vi "test_get_target_from_id.vi"() -> ()   [LabVIEW 2019]
uses:
  <vilib>/Rock Robotics/WPI/ThirdParty/PhotonVisionLib/TypeDef/PhotonTrackedTargetType.ctl
  <vilib>/Rock Robotics/WPI/ThirdParty/PhotonVisionLib/TypeDef/TargetCornerType.ctl
  <vilib>/Rock Robotics/WPI/ThirdParty/JAS_Junk/TrajLib/TypeDef/TRANSFORM3D.ctl
  <vilib>/Rock Robotics/WPI/ThirdParty/JAS_Junk/TrajLib/TypeDef/TRANSLATION3D.ctl
  <vilib>/Rock Robotics/WPI/ThirdParty/JAS_Junk/TrajLib/TypeDef/ROTATION3D.ctl
  <vilib>/Rock Robotics/WPI/ThirdParty/JAS_Junk/TrajLib/TypeDef/QUATERNION.ctl
  <vilib>/Rock Robotics/WPI/ThirdParty/PhotonVisionLib/SubVI/PhotonPipelineResult_GetLatency_Millis.vi
  <vilib>/Rock Robotics/WPI/ThirdParty/PhotonVisionLib/SubVI/Packet_encode_FLT64.vi
  <vilib>/Rock Robotics/WPI/ThirdParty/PhotonVisionLib/SubVI/Packet_encode_ByteI8.vi
  <vilib>/Rock Robotics/WPI/ThirdParty/PhotonVisionLib/SubVI/PhotonTrackedTarget_Pack.vi
  <vilib>/Rock Robotics/WPI/ThirdParty/PhotonVisionLib/SubVI/PhotonMultiTargetPNPResult_pack.vi
  <vilib>/Rock Robotics/WPI/ThirdParty/PhotonVisionLib/SubVI/Packet_decode_Flt64.vi
  <vilib>/Rock Robotics/WPI/ThirdParty/PhotonVisionLib/SubVI/Packet_decode_ByteI8.vi
  <vilib>/Rock Robotics/WPI/ThirdParty/PhotonVisionLib/SubVI/PhotonTrackedTarget_Unpack.vi
  <vilib>/Rock Robotics/WPI/ThirdParty/PhotonVisionLib/SubVI/PhotonMultiTargetPNPResult_unpack.vi
  <vilib>/Rock Robotics/WPI/ThirdParty/PhotonVisionLib/SubVI/PhotonTrackedTarget_GetArea.vi
  <vilib>/Rock Robotics/WPI/ThirdParty/PhotonVisionLib/SubVI/PhotonTrackedTarget_GetBestCameraToTarget.vi
  <vilib>/Rock Robotics/WPI/ThirdParty/PhotonVisionLib/SubVI/PhotonTrackedTarget_GetMinAreaRectCorners.vi
  <vilib>/Rock Robotics/WPI/ThirdParty/PhotonVisionLib/SubVI/PhotonTrackedTarget_GetPitch.vi
  <vilib>/Rock Robotics/WPI/ThirdParty/PhotonVisionLib/SubVI/PhotonTrackedTarget_GetSkew.vi
  <vilib>/Rock Robotics/WPI/ThirdParty/PhotonVisionLib/SubVI/PhotonTrackedTarget_GetYaw.vi
  <vilib>/Rock Robotics/WPI/ThirdParty/PhotonVisionLib/SubVI/PhotonTrackedTarget_GetAltCameraToTarget.vi
  <vilib>/Rock Robotics/WPI/ThirdParty/PhotonVisionLib/SubVI/Packet_encode_Transform3d.vi
  <vilib>/Rock Robotics/WPI/ThirdParty/PhotonVisionLib/SubVI/PhotonTrackedTarget_GetFiducialId.vi
  <vilib>/Rock Robotics/WPI/ThirdParty/PhotonVisionLib/SubVI/Packet_encode_Int32.vi
  <vilib>/Rock Robotics/WPI/ThirdParty/PhotonVisionLib/SubVI/PhotonTrackedTarget_GetPoseAmbiguity.vi
  <vilib>/Rock Robotics/WPI/ThirdParty/PhotonVisionLib/SubVI/PhotonTrackedTarget_GetDetectedCorners.vi
  <vilib>/Rock Robotics/WPI/ThirdParty/PhotonVisionLib/SubVI/PhotonPNPResult_pack.vi
  <vilib>/Rock Robotics/WPI/ThirdParty/PhotonVisionLib/SubVI/Packet_encode_Int16.vi
  <vilib>/Rock Robotics/WPI/ThirdParty/PhotonVisionLib/SubVI/PhotonMultiTargetPNPResult_MAX_IDS.vi
  <vilib>/Rock Robotics/WPI/ThirdParty/PhotonVisionLib/SubVI/TargetCorner_New.vi
  <vilib>/Rock Robotics/WPI/ThirdParty/PhotonVisionLib/SubVI/Packet_decode_Int32.vi
  <vilib>/Rock Robotics/WPI/ThirdParty/PhotonVisionLib/SubVI/Packet_decode_Transform3d.vi
  <vilib>/Rock Robotics/WPI/ThirdParty/PhotonVisionLib/SubVI/PhotonPNPResult_unpackt.vi
  <vilib>/Rock Robotics/WPI/ThirdParty/PhotonVisionLib/SubVI/PhotonMultiTargetPNPResult_New.vi
  <vilib>/Rock Robotics/WPI/ThirdParty/PhotonVisionLib/SubVI/Packet_decode_Int16.vi
  <vilib>/Rock Robotics/WPI/ThirdParty/JAS_Junk/TrajLib/VI/Transform3d_GetRotation3d.vi
  <vilib>/Rock Robotics/WPI/ThirdParty/JAS_Junk/TrajLib/VI/Transform3d_GetTranslation3d.vi
  <vilib>/Rock Robotics/WPI/ThirdParty/JAS_Junk/TrajLib/VI/Translation3d_ToTranslation2d.vi
  <vilib>/Rock Robotics/WPI/ThirdParty/JAS_Junk/TrajLib/VI/Rotation3d_ToRotation2d.vi
  <vilib>/Rock Robotics/WPI/ThirdParty/JAS_Junk/TrajLib/Transform2d_Create_TransRot.vi
  <vilib>/Rock Robotics/WPI/ThirdParty/JAS_Junk/TrajLib/VI/Transform3d_GetXYZ.vi
  <vilib>/Rock Robotics/WPI/ThirdParty/JAS_Junk/TrajLib/VI/Rotation3d_GetQuaterion.vi
  <vilib>/Rock Robotics/WPI/ThirdParty/JAS_Junk/TrajLib/VI/Quaternion_Get_All.vi
  <vilib>/Rock Robotics/WPI/ThirdParty/PhotonVisionLib/SubVI/Packet_encode_Boolean.vi
  <vilib>/Rock Robotics/WPI/ThirdParty/JAS_Junk/TrajLib/VI/Transform3d_Create_Trans3dRot3d.vi
  <vilib>/Rock Robotics/WPI/ThirdParty/JAS_Junk/TrajLib/VI/Translation3d_Create.vi
  <vilib>/Rock Robotics/WPI/ThirdParty/JAS_Junk/TrajLib/VI/Rotation3d_Create_Quaternion.vi
  <vilib>/Rock Robotics/WPI/ThirdParty/JAS_Junk/TrajLib/VI/Quaternion_New.vi
  <vilib>/Rock Robotics/WPI/ThirdParty/PhotonVisionLib/SubVI/Packet_decode_Boolean.vi
  <vilib>/Rock Robotics/WPI/ThirdParty/PhotonVisionLib/SubVI/PhotonPNPResult_New_Empty.vi
  <vilib>/Rock Robotics/WPI/ThirdParty/PhotonVisionLib/SubVI/PhotonPNPResult_New.vi
  <vilib>/Rock Robotics/WPI/ThirdParty/JAS_Junk/TrajLib/Translation2d_Create.vi
  <vilib>/Rock Robotics/WPI/ThirdParty/JAS_Junk/TrajLib/Rotation2d_CreateAngle.vi
  <vilib>/Rock Robotics/WPI/ThirdParty/JAS_Junk/TrajLib/VI/Rotation3d_GetXYZ.vi
  <vilib>/Rock Robotics/WPI/ThirdParty/JAS_Junk/TrajLib/VI/Translation3d_GetXYZ.vi
  <vilib>/Rock Robotics/WPI/ThirdParty/JAS_Junk/TrajLib/VI/Quaternion_Normalize.vi
  <vilib>/Rock Robotics/WPI/ThirdParty/JAS_Junk/TrajLib/VI/Quaternion_New_Default.vi
  <vilib>/Rock Robotics/WPI/ThirdParty/PhotonVisionLib/PhotonVisionLib.lvlib
  <vilib>/Rock Robotics/WPI/ThirdParty/JAS_Junk/TrajLib/Trajectory_Library.lvlib
panel:
  out "Target Index":i32
  out "Found Target?":bool
  out "PhotonTrackedTarget":T1={"Yaw"=0.0, "Pitch"=0.0, "Area"=0.0, "Skew"=0.0, "MinAreaRectCorners"=[], "BestCameraToTarget"={"TRANSLATION3D"={"X"=0.0, "Y"=0.0, "Z"=0.0}, "ROTATION3D"={"Q_quaternion"={"R"=1.0, "V"=[0.0, 0.0, 0.0]}}, "XF"=FALSE}, "FiiducialId"=0, "AltCameraToTarget"={"TRANSLATION3D"={"X"=0.0, "Y"=0.0, "Z"=0.0}, "ROTATION3D"={"Q_quaternion"={"R"=0.0, "V"=[0.0, 0.0, 0.0]}}, "XF"=FALSE}, "PoseAmbiguity"=0.0, "DetectedCorners"=[]} {"AltCameraToTarget"."TRANSLATION3D"."Z" format="%14.3f"; "AltCameraToTarget"."TRANSLATION3D"."Y" format="%14.3f"; "AltCameraToTarget"."TRANSLATION3D"."X" format="%14.3f"; "BestCameraToTarget"."TRANSLATION3D"."Z" format="%14.3f"; "BestCameraToTarget"."TRANSLATION3D"."Y" format="%14.3f"; "BestCameraToTarget"."TRANSLATION3D"."X" format="%14.3f"}
  in  "ID":i32
  in  "TrackedTargets":T1[](array[typedef]) {"AltCameraToTarget"."TRANSLATION3D"."Z" format="%14.3f"; "AltCameraToTarget"."TRANSLATION3D"."Y" format="%14.3f"; "AltCameraToTarget"."TRANSLATION3D"."X" format="%14.3f"; "BestCameraToTarget"."TRANSLATION3D"."Z" format="%14.3f"; "BestCameraToTarget"."TRANSLATION3D"."Y" format="%14.3f"; "BestCameraToTarget"."TRANSLATION3D"."X" format="%14.3f"}
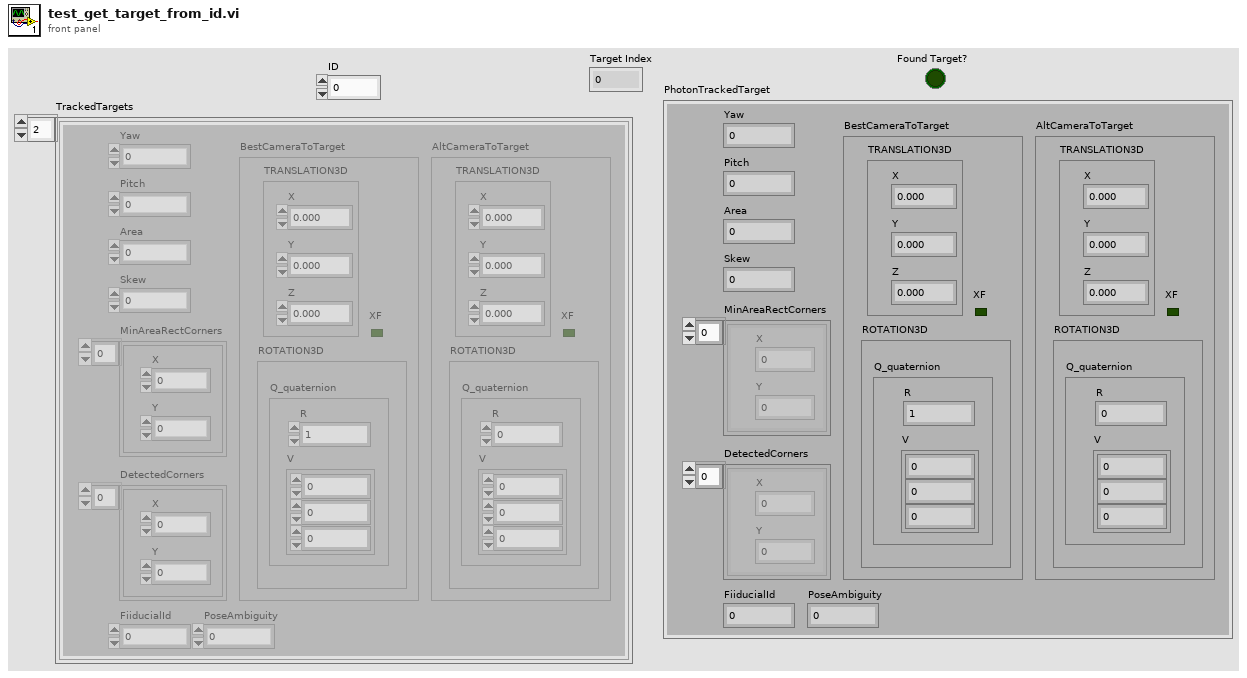
[diagram p1: front panel]
types:
  T1 = typedef "PhotonVisionLib.lvlib/PhotonTrackedTargetType.ctl" = cluster{"Yaw":dbl, "Pitch":dbl, "Area":dbl, "Skew":dbl, "MinAreaRectCorners":T2[], "BestCameraToTarget":T3, "FiiducialId":i32, "AltCameraToTarget":T3, "PoseAmbiguity":dbl, "DetectedCorners":T2[]}
  T2 = typedef "PhotonVisionLib.lvlib/TargetCornerType.ctl" = cluster{"X":dbl, "Y":dbl}
  T3 = typedef "Trajectory_Library.lvlib/TRANSFORM3D.ctl" = cluster{"TRANSLATION3D":T4, "ROTATION3D":T5, "XF":bool}
  T4 = typedef "Trajectory_Library.lvlib/TRANSLATION3D.ctl" = cluster{"X":dbl, "Y":dbl, "Z":dbl}
  T5 = typedef "Trajectory_Library.lvlib/ROTATION3D.ctl" = cluster{"Q_quaternion":T6}
  T6 = typedef "Trajectory_Library.lvlib/QUATERNION.ctl" = cluster{"R":dbl, "V":dbl[]}
  T7 = typedef "PhotonVisionLib.lvlib/PhotonPipelineResultType.ctl" = cluster{"TargetCount":i32, "Latency_MilliSec":dbl, "Targets":T1[], "TimeStampSec":dbl, "PhotonMultiTargetPNPResult":T8}
  T8 = typedef "PhotonVisionLib.lvlib/PhotonMultiTargetPNPResultType.ctl" = cluster{"PhotonPNPResult":T9, "FiducialIDsUsed":i16[]}
  T9 = typedef "PhotonVisionLib.lvlib/PhotonPNPResultType.ctl" = cluster{"IsPresent":bool, "bestReprojErr":dbl, "altReprojErr":dbl, "ambiguity":dbl, "Best":T3, "Alt":T3}
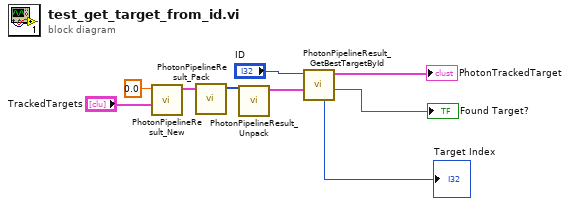
[diagram p0: block diagram]
diagram:
  n1 = call <vilib>:"PhotonPipelineResult_New.vi"("TrackedTargets"="TrackedTargets", "Latency_Millis"=0.0) -> ("PhotonPipelineResult"=w7:T7)  [unwired: 9 in]
  n2 = call <vilib>:"PhotonPipelineResult_Pack.vi"("PhotonPipelineResult"=w7) -> ("Packet_RawData"=w6:u8[])  [unwired: 10 in]
  n3 = call <vilib>:"PhotonPipelineResult_Unpack.vi"("RawData"=w6) -> ("PhotonPipelineResult"=w4:T7)  [unwired: 10 in]
  n4 = call <vilib>:"PhotonPipelineResult_GetBestTargetById.vi"("PhotonPipelineResult"=w4, "FiducialId"="ID") -> ("Target Found"=→"Found Target?":bool, "PhotonTrackedTarget"=→"PhotonTrackedTarget":T1, "Target Index"=→"Target Index":i32)  [unwired: 7 in]
